vi "Time Match.vi"(8 "Time Target":dbl, 10 "Random Second":dbl, 11 "Elapsed Time (s)":dbl) -> (1 "Elapsed Rounded":dbl, 2 "Matched?":bool, 3 "Time Left":i32)   [LabVIEW 2018, in "CollectionSupport.lvlib"]
uses:
  CollectionSupport.lvlib
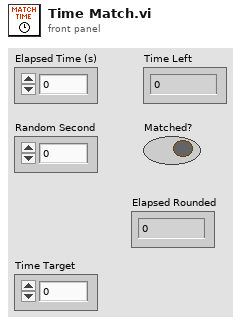
[diagram p1: front panel]
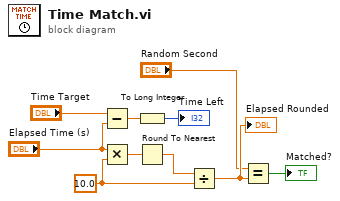
[diagram p0: block diagram]
diagram:
  w2 = 10.0 ("x")
  n1 = Subtract(x="Time Target", y="Elapsed Time (s)") -> (x-y=w7:dbl)
  n2 = Multiply(x="Elapsed Time (s)", y=w2) -> (x*y=w8:dbl)
  n3 = To Long Integer(number=w7) -> (32bit integer=→"Time Left":i32)
  n4 = Round To Nearest(number=w8) -> (nearest integer value=w9:dbl)
  n5 = Divide(x=w9, y=w2) -> (x/y=w10:dbl)
  "Elapsed Rounded" <- w10
  n6 = Equal?(x="Random Second", y=w10) -> (x = y?=→"Matched?":bool)
